vi "Compute 2D Rotation Affine Matrix.vi"(2 "Scale (Default: 1)":dbl=1.0, 3 "Angle (Deg)":dbl, 4 "Rotate Around (Default: 0,0)":T2) -> (0 "2D Affine Rotation Matrix":T1)   [LabVIEW 2020, in "image.lvlib"]
uses:
  image.lvlib
  common/Image Point (Float).ctl
  <vilib>/Analysis/Matrix/Datatypes/RealMatrix.ctl
  <vilib>/Analysis/Matrix/NI_Matrix.lvlib
  common/common.lvlib
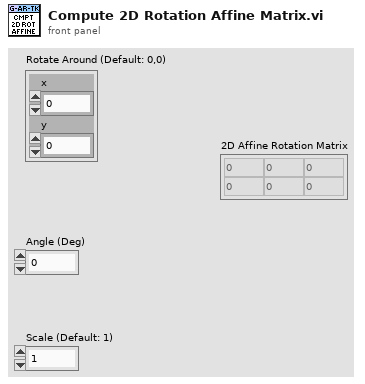
[diagram p1: front panel]
types:
  T1 = typedef "NI_Matrix.lvlib/RealMatrix.ctl" = dbl[][]
  T2 = typedef "common.lvlib/Image Point (Float).ctl" = cluster{"x":dbl, "y":dbl}
  T3 = cluster{"alpha":dbl, "beta":dbl, "(1-alpha)":dbl, "-beta":dbl}
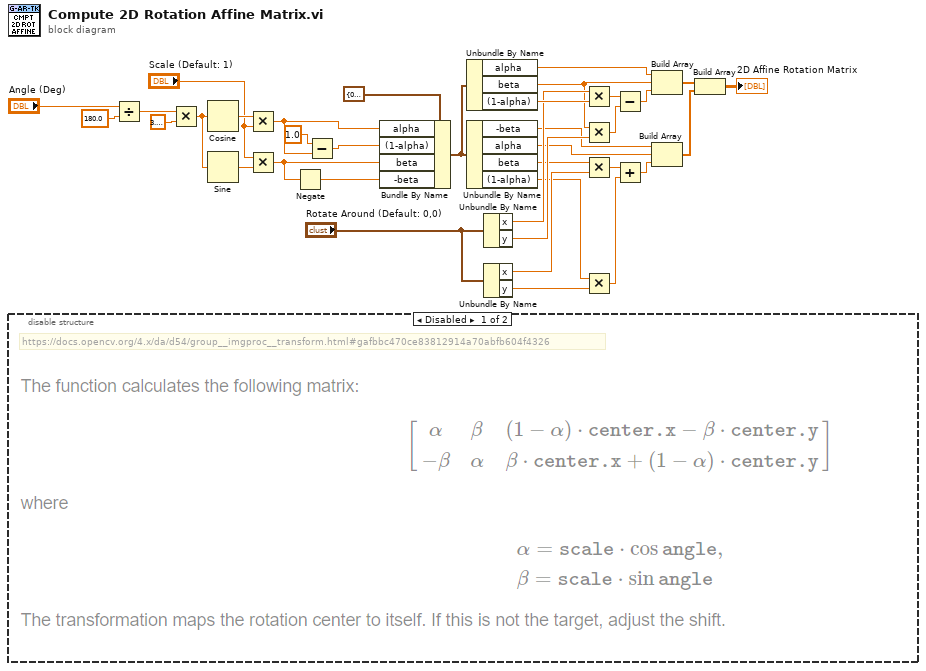
[diagram p0: block diagram]
diagram:
  n1 = disable-structure shown="Disabled" {
    frame Disabled {
      # "https://docs.opencv.org/4.x/da/d54/group__imgproc__transform.html#gafbbc470ce83812914a70abfb604f4326"
    }
    frame Enabled {
    }
  }
  n2 = Divide(x="Angle (Deg)", y=180.0 ("x")) -> (x/y=w6:dbl)
  n3 = Multiply(x=w6, y=3.141592653589793) -> (x*y=w4:dbl)
  n4 = Cosine(x=w4) -> (cos(x)=w34:dbl)
  n5 = Sine(x=w4) -> (sin(x)=w35:dbl)
  n6 = Multiply(x=w34, y="Scale (Default: 1)") -> (x*y=w31:dbl)
  n7 = Multiply(x="Scale (Default: 1)", y=w35) -> (x*y=w1:dbl)
  n8 = Negate(x=w1) -> (-x=w21:dbl)
  n9 = Subtract(x=1.0, y=w31) -> (x-y=w2:dbl)
  n10 = Bundle By Name(cluster=T3 {"alpha"=0.0, "beta"=0.0, "(1-alpha)"=0.0, "-beta"=0.0} ("output cluster"), "alpha"=w31, "(1-alpha)"=w2, "beta"=w1, "-beta"=w21) -> (w20:T3)
  n11 = Unbundle By Name(w20) -> ("alpha"=w22:dbl, "beta"=w23:dbl, "(1-alpha)"=w29:dbl)
  n12 = Unbundle By Name(w20) -> ("-beta"=w19:dbl, "alpha"=w18:dbl, "beta"=w16:dbl, "(1-alpha)"=w12:dbl)
  n13 = Unbundle By Name("Rotate Around (Default: 0,0)") -> ("x"=w28:dbl, "y"=w27:dbl)
  n14 = Unbundle By Name("Rotate Around (Default: 0,0)") -> ("x"=w15:dbl, "y"=w13:dbl)
  n15 = Multiply(x=w28, y=w29) -> (x*y=w26:dbl)
  n16 = Multiply(x=w23, y=w27) -> (x*y=w25:dbl)
  n17 = Multiply(x=w16, y=w15) -> (x*y=w14:dbl)
  n18 = Multiply(x=w12, y=w13) -> (x*y=w11:dbl)
  n19 = Subtract(x=w26, y=w25) -> (x-y=w24:dbl)
  n20 = Add(x=w14, y=w11) -> (x+y=w10:dbl)
  n21 = Build Array(w22, w23, w24) -> (w9:dbl[])
  n22 = Build Array(w19, w18, w10) -> (w8:dbl[])
  n23 = Build Array(w9, w8) -> (→"2D Affine Rotation Matrix":T1)
